vi "MakeButtonVerySmall.vi"(8 "error in (no error)":errorcluster, 10 "visible":bool, 11 "Link Button 1":refnum<vi>) -> (0 "error out":errorcluster, 3 "Link Button 2":refnum<vi>)   [LabVIEW 2009, in "NavScreen.lvlib"]
uses:
  NavScreen.lvlib
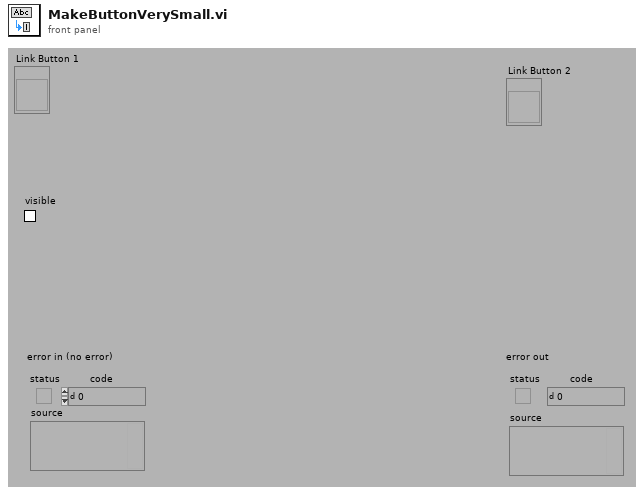
[diagram p1: front panel]
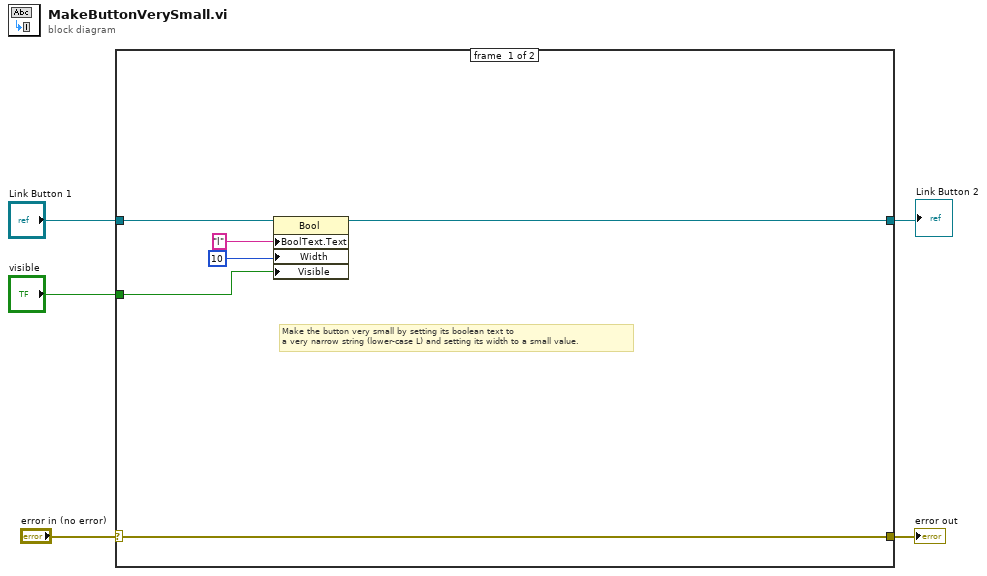
[diagram p0: block diagram]
diagram:
  n1 = case shown="No Error" "error in (no error)" {
    selector: "error in (no error)" -> [w11 w13]
    tunnel: [w11 w13] -> w4
    tunnel: "visible" -> [w7 _]
    tunnel: "Link Button 1" -> [w8 w12]
    tunnel: [w6 w12] -> w1
    frame #0 {
      # "Make the button very small by setting its boolean text to \na very narrow string (lower-case L) and setting its width to a small value."
      n2 = property class="Bool"(reference=w8, "BoolText.Text"="l" ("Boolean Text.Text"), "Width"=u32 10 ("Button Size:Width"), "Visible"=w7) -> (reference out=w6:refnum<vi>)  [unwired: 1 in, 1 out]
    }
    frame #1 {
    }
  }
  "error out" <- w4
  "Link Button 2" <- w1
